vi "stopMotion.vi"(8 "error in (no error)":errorcluster, 10 "model":refnum<class "Model.lvclass">, 11 "ControlledMotionState in":refnum<class "ControlledMotionState.lvclass">) -> (0 "error out":errorcluster, 2 "model 2":refnum<class "Model.lvclass">, 3 "ControlledMotionState out":refnum<class "ControlledMotionState.lvclass">)   [LabVIEW 2013, in "ControlledMotionState.lvclass"]
uses:
  ControlledMotionState.lvclass
  Model/Model/Model.lvclass
  Typedefs/StateSelector.ctl
  EnabledState/EnabledState.lvclass
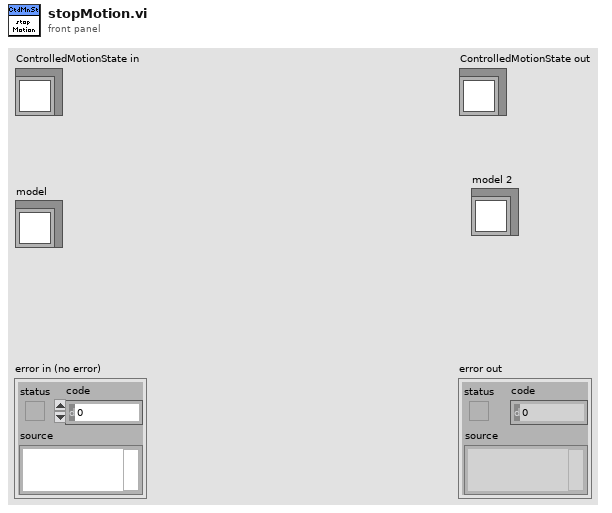
[diagram p1: front panel]
types:
  T1 = typedef "StateSelector.ctl" = enum16{"EndingCycleState", "FaultState", "InteractiveMotionState", "MovingToNewForceState", "OffState", "PausingState", "StandbyState", "StoppedState"}
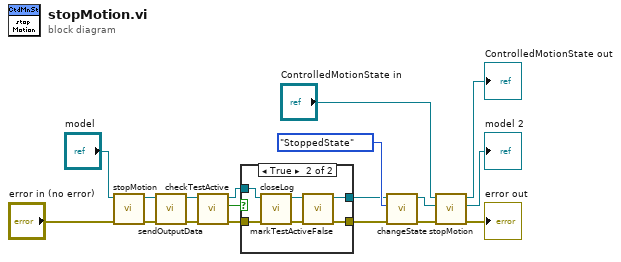
[diagram p0: block diagram]
diagram:
  n1 = call "stopMotion.vi"("error in (no error)"="error in (no error)", "Model in"="model") -> ("error out"=w2:errorcluster, "Model out"=w4:refnum<class "Model.lvclass">)  [unwired: 8 in]
  n2 = call "sendOutputData.vi"("error in (no error)"=w2, "Model in"=w4) -> ("error out"=w1:errorcluster, "Model out"=w3:refnum<class "Model.lvclass">)  [unwired: 8 in]
  n3 = call "checkTestActive.vi"("error in (no error)"=w1, "Model in"=w3) -> ("error out"=w5:errorcluster, "testActiveIsTrue"=w7:bool, "Model out"=w6:refnum<class "Model.lvclass">)  [unwired: 7 in]
  n4 = case shown="True" w7 {
    tunnel: [w20 w23] -> w9
    tunnel: [w19 w21] -> w8
    tunnel: w6 -> [w20 w26]
    tunnel: w5 -> [w19 w25]
    frame False {
    }
    frame True {
      n5 = call "closeLog.vi"("error in (no error)"=w25, "Model in"=w26) -> ("error out"=w22:errorcluster, "Model out"=w24:refnum<class "Model.lvclass">)  [unwired: 8 in]
      n6 = call "markTestActiveFalse.vi"("error in (no error)"=w22, "Model in"=w24) -> ("error out"=w21:errorcluster, "Model out"=w23:refnum<class "Model.lvclass">)  [unwired: 8 in]
    }
  }
  n7 = call "changeState.vi"("error in (no error)"=w8, "State:"=StateSelector."StoppedState", "Model in"=w9) -> ("error out"=w11:errorcluster, "Model out"=w13:refnum<class "Model.lvclass">)  [unwired: 7 in]
  n8 = call-parent "stopMotion.vi"("error in (no error)"=w11, "model"=w13, "State in"="ControlledMotionState in") -> ("error out"=→"error out":errorcluster, "model 2"=→"model 2":refnum<class "Model.lvclass">, "State out"=→"ControlledMotionState out":refnum<class "ControlledMotionState.lvclass">)  [unwired: 6 in]
